vi "Set Connection.vi"(5 "Server Port Type":enum8{"CMD", "TLM", "BOTH"}(ring), 7 "Server Port":u16, 8 "Client":refnum<k5>, 9 "Client Port":u16, 10 "Client IP":string, 11 "Connection in":refnum<data-value>) -> (0 "error out":errorcluster, 3 "Connection out":refnum<data-value>)   [LabVIEW 2018, in "TCPServer.lvlib"]
uses:
  TCPServer.lvlib
  TypeDefs/Connection.ctl
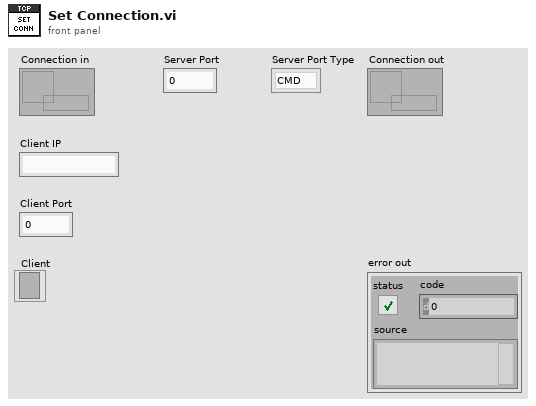
[diagram p1: front panel]
types:
  T1 = typedef "TCPServer.lvlib/Connection.ctl" = cluster{"Tcp":refnum<k5>, "Server Port":u16, "Server Port Type":enum8{"CMD", "TLM", "BOTH"}, "Client IP":string, "Client Port":u16}
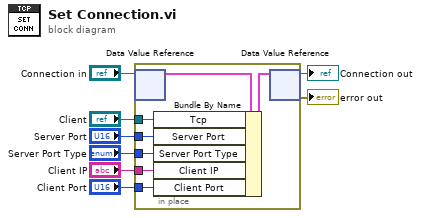
[diagram p0: block diagram]
diagram:
  n1 = in-place {
    in-place-border: "Client" -> [w13]
    in-place-border: "Server Port" -> [w12]
    in-place-border: "Server Port Type" -> [w11]
    in-place-border: "Client IP" -> [w10]
    in-place-border: "Client Port" -> [w9]
    n2 = in-place-dvr #1("Connection in") -> (w15:T1)  [unwired: 1 out]
    n3 = Bundle By Name(cluster=w15, "Tcp"=w13, "Server Port"=w12, "Server Port Type"=w11, "Client IP"=w10, "Client Port"=w9) -> (w14:T1)
    n4 = in-place-dvr #1(w14) -> (→"Connection out":refnum<data-value>, →"error out":errorcluster)
  }
